vi "Update Channel.vi"(8 "error in (no error)":errorcluster, 9 "Channel Index":i32, 10 "Channel":refnum<class "Channel.lvclass">, 11 "SignalManager in":refnum<class "SignalManager.lvclass">) -> (0 "error out":errorcluster, 3 "SignalManager out":refnum<class "SignalManager.lvclass">)   [LabVIEW 2015, in "SignalManager.lvclass"]
uses:
  SignalManager.lvclass
  Channel/Channel.lvclass
  SignalManager.lvclass/SignalManager.ctl
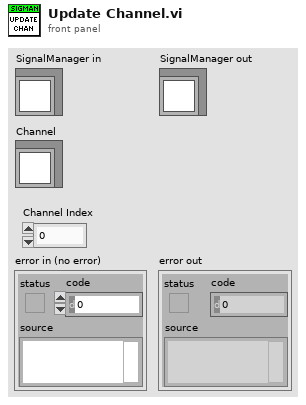
[diagram p1: front panel]
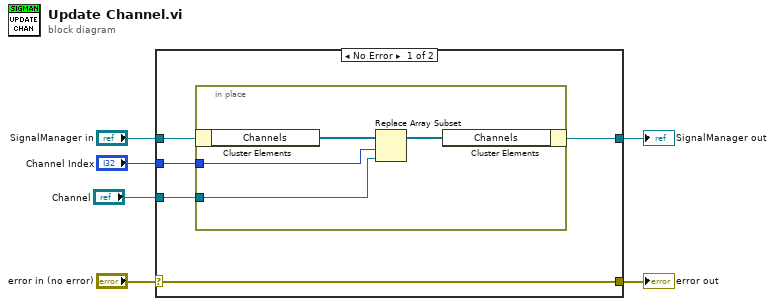
[diagram p0: block diagram]
diagram:
  n1 = case shown="No Error" "error in (no error)" {
    selector: "error in (no error)" -> [w11 w17]
    tunnel: [w11 w17] -> w5
    tunnel: [w9 w16] -> w3
    tunnel: "SignalManager in" -> [w10 w16]
    tunnel: "Channel Index" -> [w8 _]
    tunnel: "Channel" -> [w7 _]
    frame No Error {
      n2 = in-place {
        in-place-border: w8 -> [w13]
        in-place-border: w7 -> [w12]
        n3 = in-place-cluster #1(w10) -> ("Channels"=w15:refnum<class "Channel.lvclass">[])
        n4 = Replace Array Subset(array=w15, new element=w12, index=w13) -> (w14:refnum<class "Channel.lvclass">[])
        n5 = in-place-cluster #1("Channels"=w14) -> (w9:refnum<class "SignalManager.lvclass">)
      }
    }
    frame Error {
    }
  }
  "error out" <- w5
  "SignalManager out" <- w3
